vi "Begin.vi"(8 "error in (no error)":errorcluster, 11 "Comp Motors with Brake in":refnum<class "Comp Motors with Brake.lvclass">) -> (0 "error out":errorcluster, 3 "Comp Motors with Brake out":refnum<class "Comp Motors with Brake.lvclass">)   [LabVIEW 2014, in "Comp Motors with Brake.lvlib" / "Comp Motors with Brake.lvclass"]
uses:
  Comp Motors with Brake.lvclass
  Comp Motors with Brake.lvclass/Comp Motors with Brake.ctl
  <vilib>/Rock Robotics/WPI/Solenoid/WPI_SolenoidOpenSingle.vi
  Comp Motors with Encoders/Comp Motors with Encoders Class/Comp Motors with Encoders.lvclass
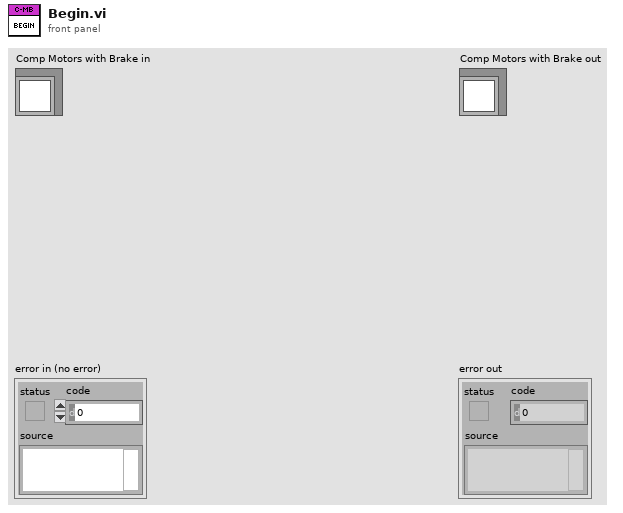
[diagram p1: front panel]
types:
  T1 = typedef "WPI_SolenoidChannel.ctl" = enum8{"Solenoid 0", "Solenoid 1", "Solenoid 2", "Solenoid 3", "Solenoid 4", "Solenoid 5", "Solenoid 6", "Solenoid 7", "Invalid"}
  T2 = typedef "WPI_SolenoidDevRef.ctl" = cluster{"DevStatus":errorcluster, "Pneumatics Control Module":u8, "Forward Solenoid Channel":T1, "Reverse Solenoid Channel":T1}
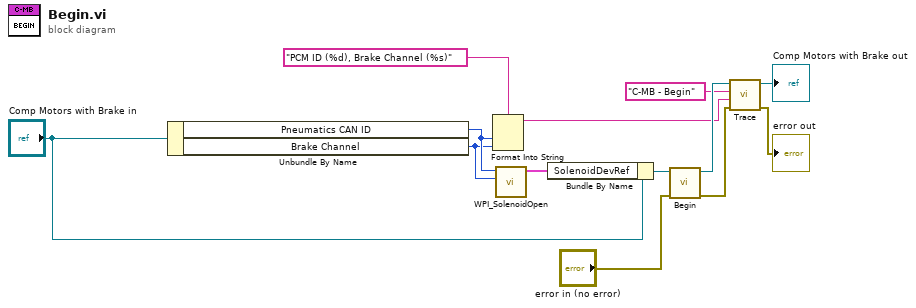
[diagram p0: block diagram]
diagram:
  n1 = Unbundle By Name("Comp Motors with Brake in") -> ("Pneumatics CAN ID"=w3:u8, "Brake Channel"=w2:T1)
  n2 = Format Into String(format string="PCM ID (%d), Brake Channel (%s)", w3, w2) -> (resulting string=w1:string)  [unwired: 2 in, 1 out]
  n3 = call-poly <vilib>:"WPI_SolenoidOpen.vi"("Solenoid Channel"=w2, "Pneumatics Control Module (0)"=w3) -> ("SolenoidDevRef"=w10:T2)  [unwired: 8 in, 1 out]
  n4 = Bundle By Name(cluster="Comp Motors with Brake in", "SolenoidDevRef"=w10) -> (w11:refnum<class "Comp Motors with Brake.lvclass">)
  n5 = call-parent "Begin.vi"("error in (no error)"="error in (no error)", "Comp Motors with Encoders in"=w11) -> ("error out"=w7:errorcluster, "Comp Motors with Encoders out"=w9:refnum<class "Comp Motors with Brake.lvclass">)  [unwired: 8 in]
  n6 = call-dynamic "Trace.vi"("error in (no error)"=w7, "System Message"=w1, "System Action"="C-MB - Begin", "System Actor in"=w9) -> ("error out"=→"error out":errorcluster, "System Actor out"=→"Comp Motors with Brake out":refnum<class "Comp Motors with Brake.lvclass">)  [unwired: 6 in]
